vi "Get Log Text Array From Log File.vi"(8 "error in":errorcluster, 11 "Log File Path in":path) -> (0 "error out":errorcluster, 2 "Log Text Array":string[](array[string]), 3 "Log File Path out":path)   [LabVIEW 2020, in "Testing.lvlib"]
uses:
  Testing.lvlib
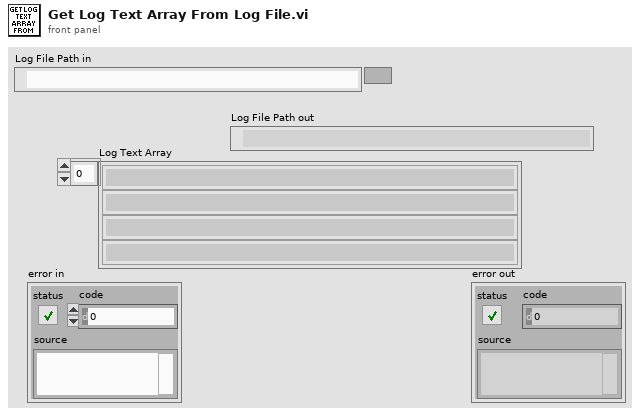
[diagram p1: front panel]
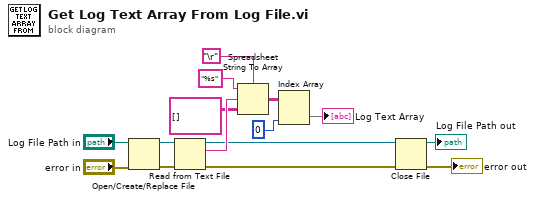
[diagram p0: block diagram]
diagram:
  n1 = Open/Create/Replace File(file path (use dialog)="Log File Path in", error in="error in") -> (refnum out=w5:refnum<file>, error out=w4:errorcluster)  [unwired: 4 in, 1 out]
  n2 = Read from Text File(file (use dialog)=w5, error in=w4) -> (refnum out=w7:refnum<file>, text=w12:string, error out=w6:errorcluster)  [unwired: 2 in, 1 out]
  n3 = Spreadsheet String To Array(delimiter (Tab)="\r", format string="%s", spreadsheet string=w12, array type (2D Dbl)=string[][] []) -> (array=w13:string[][])
  n4 = Index Array(array=w13, index (col)=0 ("disabled index (col)")) -> (element=→"Log Text Array":string[])  [unwired: 1 in]
  n5 = Close File(refnum=w7, error in=w6) -> (path=→"Log File Path out":path, error out=→"error out":errorcluster)
